vi "_Kaelus PIM Tree.vi"   [LabVIEW 2011]
uses:
  PIM Command.ctl
panel:
  # "Kaelus PIM Driver Tree\nSee Diagram"
types:
  T1 = typedef "PIM Command.ctl" = enum16{"LOAD", "KEEP ALIVE", "VALIDATE", "INITIALIZE", "PRESET", "GET CALIBRATION", "SET STIMULUS", "TOGGLE TX POWER", "SET TX ON", "SET TX OFF", "MEASURE", "UNLOAD"}
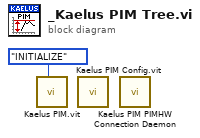
[diagram p0: block diagram]
diagram:
  n1 = call "Kaelus PIM.vit"("PIM Command"=PIM_Command."INITIALIZE") -> ()  [unwired: 3 in, 8 out]
  n2 = call "Kaelus PIM Config.vit"() -> ()  [unwired: 2 in, 10 out]
  n3 = call "Kaelus PIM PIMHW Connection Daemon.vi"() -> ()  [unwired: 1 in, 11 out]
